vi "Add Client.vi"(8 "error in (no error)":errorcluster, 9 "Client ID":string, 10 "WebSocket Connection":refnum<k5>, 11 "WebSocket Service Actor in":refnum<class "WebSocket Service Actor.lvclass">) -> (0 "error out":errorcluster, 3 "WebSocket Service Actor out":refnum<class "WebSocket Service Actor.lvclass">)   [LabVIEW 2016, in "WebSocket Actor.lvlib" / "WebSocket Service Actor.lvclass"]
uses:
  WebSocket Service Actor.lvclass
  C:/Program Files (x86)/National Instruments/LabVIEW 2016/vi.lib/ActorFramework/Actor/Actor.lvclass
  WebSocket Connection/WebSocket Connection.lvclass
  WebSocket Connection/WebSocket Connection.lvclass/WebSocket Connection.ctl
  WebSocket Connection/properties/Write WebSocket Connection.vi
  WebSocket Connection/properties/Write Client ID.vi
  <vilib>/ActorFramework/Actor/Actor.lvclass
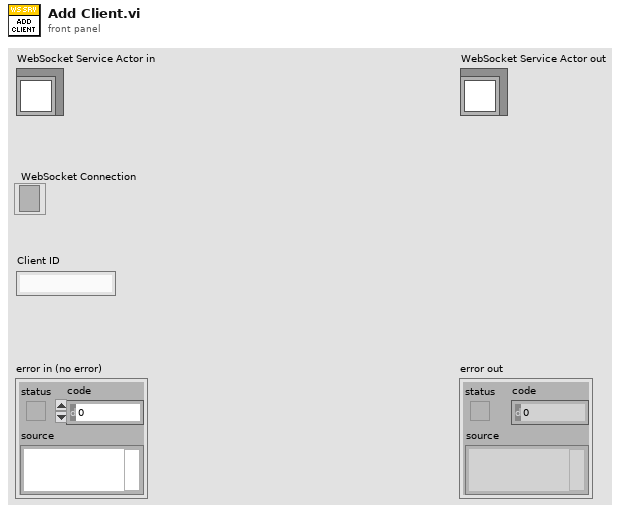
[diagram p1: front panel]
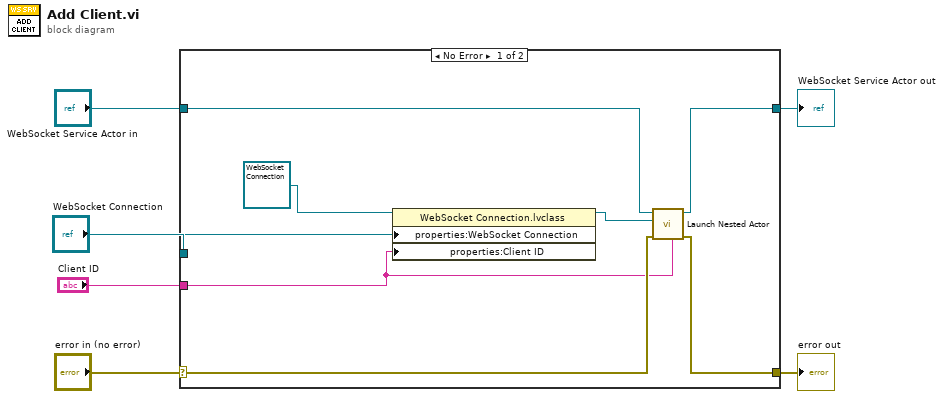
[diagram p0: block diagram]
diagram:
  n1 = case shown="No Error" "error in (no error)" {
    selector: "error in (no error)" -> [w11 w16]
    tunnel: [w10 w16] -> w5
    tunnel: [w12 w15] -> w3
    tunnel: "WebSocket Service Actor in" -> [w13 w15]
    tunnel: "WebSocket Connection" -> [w8 _]
    tunnel: "Client ID" -> [w7 _]
    frame No Error {
      n2 = property class="WebSocket Connection.lvclass"(reference=refnum<class "WebSocket Connection.lvclass"> refnum ("WebSocket Connection.lvclass"), "properties:WebSocket Connection"=w8, "properties:Client ID"=w7) -> (reference out=w14:refnum<class "WebSocket Connection.lvclass">)  [unwired: 1 in, 1 out]
      n3 = call <vilib>:"Launch Nested Actor.vi"("Debug Alias"=w7, "error in (no error)"=w11, "Nested Actor"=w14, "Caller Actor in"=w13) -> ("error out"=w10:errorcluster, "Caller Actor out"=w12:refnum<class "WebSocket Service Actor.lvclass">)  [unwired: 5 in, 1 out]
    }
    frame Error {
    }
  }
  "error out" <- w5
  "WebSocket Service Actor out" <- w3
